vi "CheckInternet.vi"(8 "error in (no error)":errorcluster) -> (0 "error out":errorcluster, 1 "Result":string, 3 "Available":bool)   [LabVIEW 2018, in "Acquisition.lvlib"]
uses:
  Acquisition.lvlib
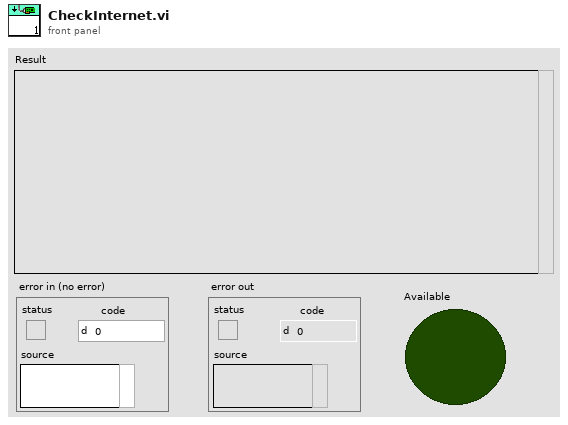
[diagram p1: front panel]
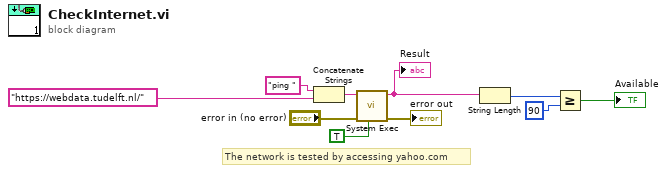
[diagram p0: block diagram]
diagram:
  # "The network is tested by accessing yahoo.com"
  n1 = Concatenate Strings("ping " ("command line"), "https://webdata.tudelft.nl/" ("PC Name or IP Address")) -> (w10:string)
  n2 = call <vilib>:"System Exec.vi"("run minimized? (F)"=TRUE, "error in (no error)"="error in (no error)", "command line"=w10) -> ("error out"=→"error out":errorcluster, "standard output"=w5:string)  [unwired: 3 in, 4 out]
  "Result" <- w5
  n3 = String Length(string=w5) -> (length=w4:i32)
  n4 = Greater Or Equal?(x=w4, y=90) -> (x >= y?=→"Available":bool)
